vi "kalman filter demo.vi"() -> ()   [LabVIEW 2014]
uses:
  <vilib>/Platform/TimedLoop/XDataNode/timing_clust.ctl
  <vilib>/Platform/TimedLoop/XDataNode/nitl_modes.ctl
  <vilib>/Platform/TimedLoop/XDataNode/wakeup.ctl
  <vilib>/Platform/TimedLoop/XDataNode/XDataNode.xnode
  <vilib>/Platform/TimedLoop/XDataNode/XDNodeRunTimeDep.lvlib
  <vilib>/ptbypt/NI_PtbyPt.lvlib
panel:
  out "Finished Late? [i-1]":bool
  out "Waveform Chart":cluster{dbl, "x_out":dbl}(graph)={7.81541398555105, "x_out"=7.299341692996249}
  in  "R":dbl=0.1
  in  "Q":dbl=1.0
  in  "stop":bool
  # "more aggressive means\nsmaller R (measurement noise covariance)\nbigger Q (process noise covariance)"
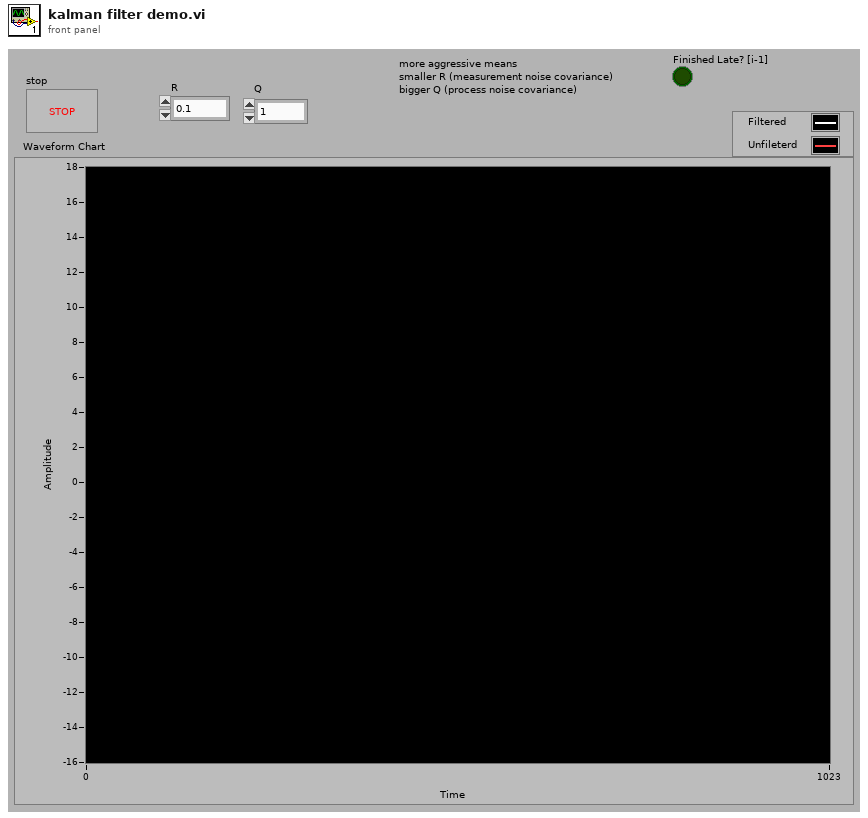
[diagram p1: front panel]
types:
  T1 = typedef "XDNodeRunTimeDep.lvlib/timing_clust.ctl" = cluster{"Expected End [f-1]":u64, "Actual End [f-1]":u64, "Finished Late? [f-1]":bool, "Expected End [i-1]":u64, "Actual End [i-1]":u64, "Finished Late? [i-1]":bool, "Expected Start [i]":u64, "Actual Start [i]":u64, "Expected Start [f]":u64, "Actual Start [f]":u64, "Source Name":string, "Structure Name":string, "Period":i64, "Deadline":i64, "Offset":i64, "Start":i64, "Priority":i32, "Timeout":i32, "Mode":T2, "Wakeup Reason":T3, "Error":errorcluster, "Source Type":string, "Secondary Source Type":string, "Global End Time":u64, "Global Start Time":u64, "Frame Duration":u64, "Iteration Duration":u64, "Assigned CPU":i32, "I/O Scan Engine Mode":u32}
  T2 = typedef "XDNodeRunTimeDep.lvlib/nitl_modes.ctl" = enum32{"No Change", "Process missed periods, maintain original phase", "Discard missed periods, maintain original phase", "Process missed periods, ignore original phase", "Discard missed periods, ignore original phase"}
  T3 = typedef "XDNodeRunTimeDep.lvlib/wakeup.ctl" = enum32{"Normal", "Aborted", "Asynchronous wakeup", "Timing source error", "Timed loop error", "Timeout"}
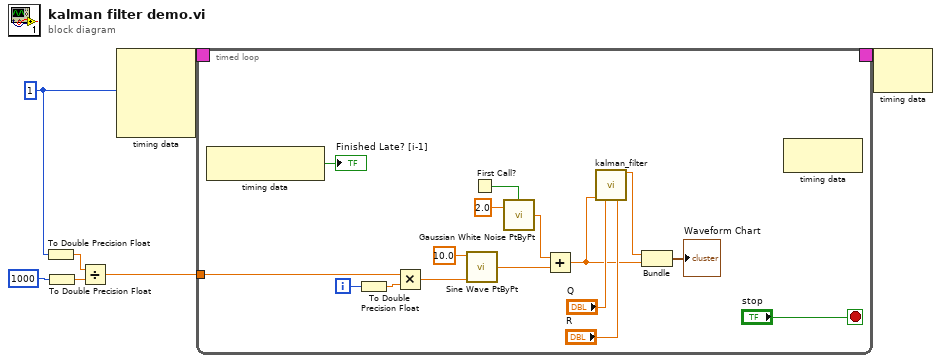
[diagram p0: block diagram]
diagram:
  w3 = i64 1 ("Period")
  n1 = To Double Precision Float(number=w3) -> (double precision float=w4:dbl)
  n2 = To Double Precision Float(number=i64 1000 ("y")) -> (double precision float=w5:dbl)
  n3 = Divide(x=w4, y=w5) -> (x/y=w1:dbl)
  n4 = node-c288(w3) -> (w7:T1)  [unwired: 3 in]
  n5 = timed-loop {
    timing: w7 -> [_]
    timing-out: [_] -> w6
    tunnel: w1 -> [w22]
    i -> [w21]
    stop <- "stop" stop-if-true
    n6 = node-c288() -> (→"Finished Late? [i-1]":bool)  [unwired: 1 in]
    n7 = To Double Precision Float(number=w21) -> (double precision float=w20:dbl)
    n8 = Multiply(x=w22, y=w20) -> (x*y=w19:dbl)
    n9 = call <vilib>:"Sine Wave PtByPt.vi"("time"=w19, "amplitude"=10.0) -> ("sine wave"=w13:dbl)  [unwired: 2 in]
    n10 = First Call?() -> (First Call?: T/F=w12:bool)
    n11 = call <vilib>:"Gaussian White Noise PtByPt.vi"("initialize"=w12, "standard deviation"=2.0) -> ("Gaussian white noise"=w17:dbl)  [unwired: 1 in]
    n12 = Add(x=w17, y=w13) -> (x+y=w10:dbl)
    n13 = call "kalman_filter.vi"("u"=w10, "Q"="Q", "R"="R") -> ("xest"=w8:dbl)  [unwired: 12 in]
    n14 = Bundle("xest"=w8, w10) -> (→"Waveform Chart":cluster{"xest":dbl, dbl})  [unwired: 1 in]
    n15 = node-c288() -> ()  [unwired: 1 in, 1 out]
  }
  n16 = node-c288(w6) -> ()  [unwired: 1 out]
